vi "Get Physcial Relay State.vi"(8 "error in (no error)":errorcluster, 10 "relay index":i32, 11 "SLSC Switch in":refnum<class "SLSC Switch.lvclass">) -> (0 "error out":errorcluster, 2 "position":T1=10 items=["Open"=10, "Closed"=11])   [LabVIEW 2015, in "SLSC Switch.lvclass"]
uses:
  SLSC Switch.lvclass
  Route Manager/Position.ctl
  SLSC Switch.lvclass/SLSC Switch.ctl
  <vilib>/SLSC/Get Device Property (Bool).vi
  <vilib>/SLSC/SLSC.lvlib
  Route Manager/Route Manager.lvclass
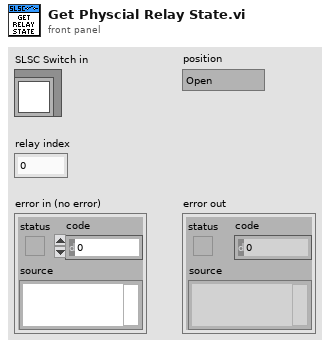
[diagram p1: front panel]
types:
  T1 = typedef "Route Manager.lvclass/Position.ctl" = i32
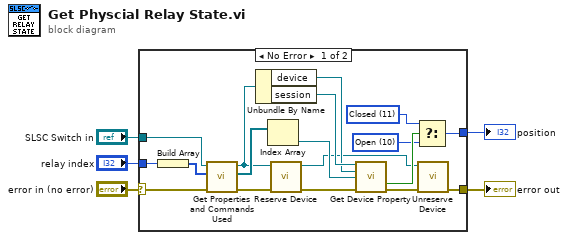
[diagram p0: block diagram]
diagram:
  n1 = case shown="No Error" "error in (no error)" {
    selector: "error in (no error)" -> [w13 w24]
    tunnel: [w6 w24] -> w4
    tunnel: "SLSC Switch in" -> [w14 _]
    tunnel: [w20 _] -> w2
    tunnel: "relay index" -> [w12 _]
    frame No Error {
      w21 = T1 11 items=["Open"=10, "Closed"=11] ("t")
      w22 = T1 10 items=["Open"=10, "Closed"=11] ("position")
      n2 = Build Array(w12) -> (w17:i32[])
      n3 = call "Get Properties and Commands Used.vi"("error in (no error)"=w13, "relays"=w17, "SLSC Switch in"=w14) -> ("error out"=w9:errorcluster, "properties"=w16:refnum<k21>[], "SLSC Switch out"=w11:refnum<class "SLSC Switch.lvclass">)  [unwired: 5 in, 1 out]
      n4 = Unbundle By Name(w11) -> ("device"=w18:refnum<k21>, "session"=w19:refnum<k21>)
      n5 = Index Array(array=w16) -> (element=w15:refnum<k21>)  [unwired: 1 in]
      n6 = call "Reserve Device.vi"("error in (no error)"=w9, "SLSC Switch in"=w11) -> ("error out"=w8:errorcluster, "SLSC Switch out"=w10:refnum<class "SLSC Switch.lvclass">)  [unwired: 8 in]
      n7 = call-poly <vilib>:"Get Device Property.vi"("session in"=w19, "devices"=w18, "property"=w15, "error in (no error)"=w8) -> ("property value"=w23:bool, "error out"=w7:errorcluster)  [unwired: 9 in, 1 out]
      n8 = Select(t=w21, s=w23, f=w22) -> (s? t:f=w20:T1)
      n9 = call "Unreserve Device.vi"("error in (no error)"=w7, "SLSC Switch in"=w10) -> ("error out"=w6:errorcluster)  [unwired: 8 in, 1 out]
    }
    frame Error {
    }
  }
  "error out" <- w4
  "position" <- w2
